vi "PR4000 cfg data.vi"(8 "error in (no error)":errorcluster, 10 "Channel parsed command info":T1, 11 "MKS4000b in":refnum<class "MKS4000b.lvclass">) -> (0 "error out":errorcluster, 2 "new commands":string, 3 "MKS4000b out":refnum<class "MKS4000b.lvclass">)   [LabVIEW 2013, in "MKS4000b.lvclass"]
uses:
  MKS4000b.lvclass
  Shared/Device Driver/channel parsed cmd cluster.ctl
  MKS4000b.lvclass/MKS4000b.ctl
  shared/CompressAndUpdate(Poly)/CompressAndUpdate(Numeric).vi
  shared/CompressAndUpdate(Poly)/CompressAndUpdate(Enum).vi
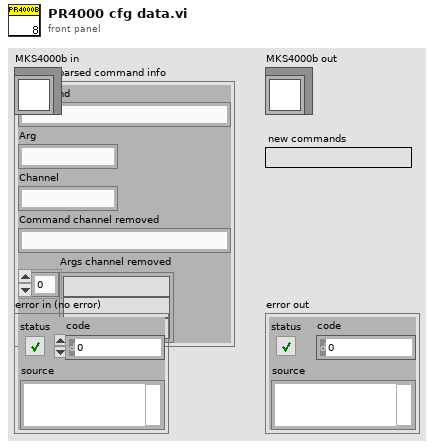
[diagram p1: front panel]
types:
  T1 = typedef "channel parsed cmd cluster.ctl" = cluster{"Command":string, "Arg":string, "Channel":string, "Command channel removed":string, "Args channel removed":string[]}
  T2 = typedef "channel_mode_typdef.ctl" = enum16{"Pressure", "Flow"}
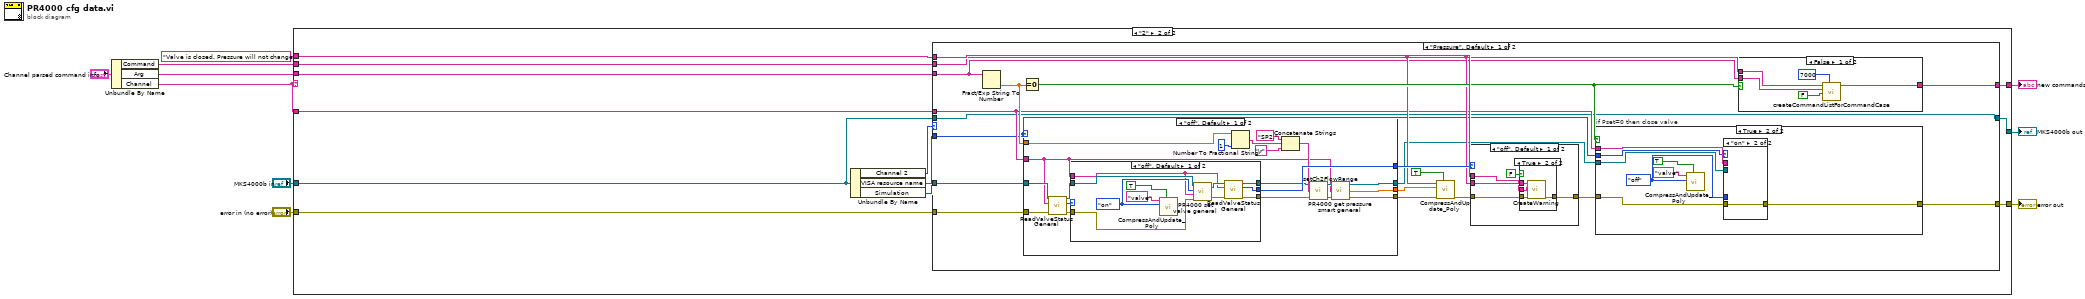
[diagram p0: block diagram]
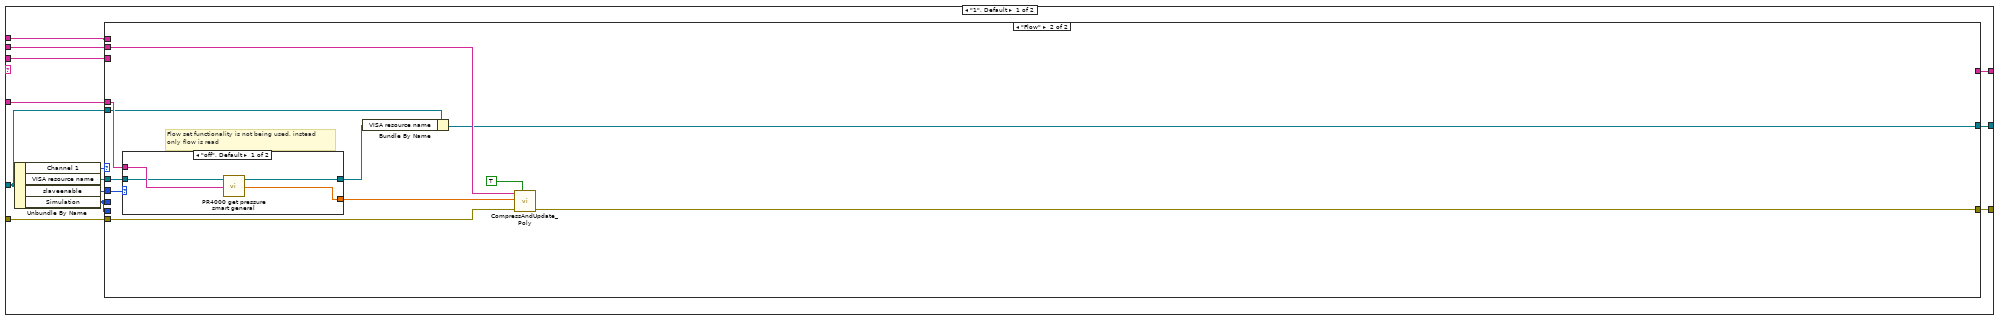
[diagram p2: hidden frame]
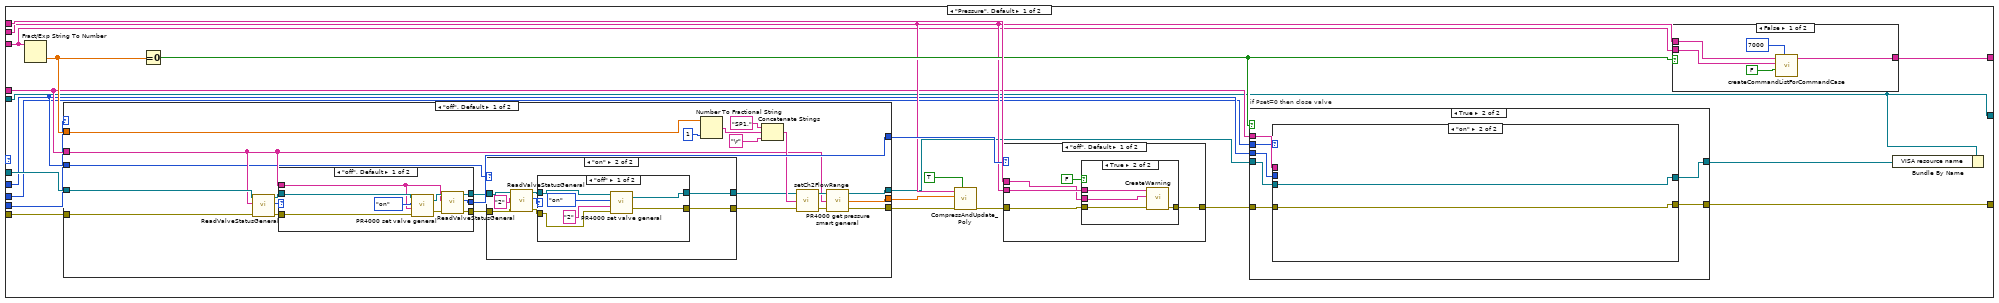
[diagram p3: hidden frame]
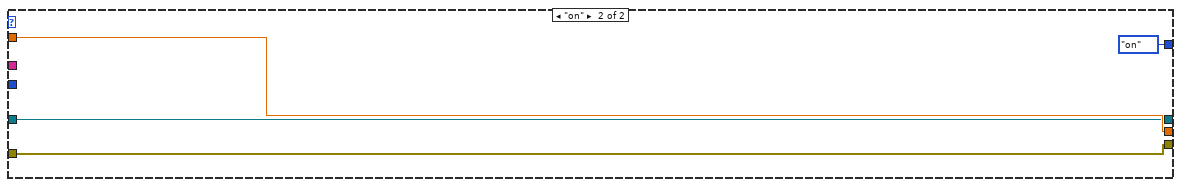
[diagram p7: hidden frame]
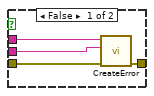
[diagram p9: hidden frame]
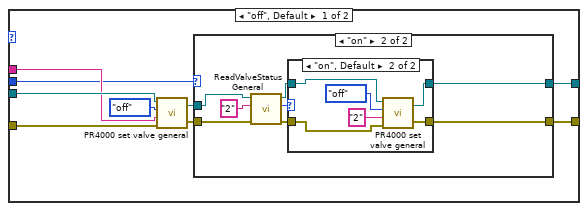
[diagram p12: hidden frame]
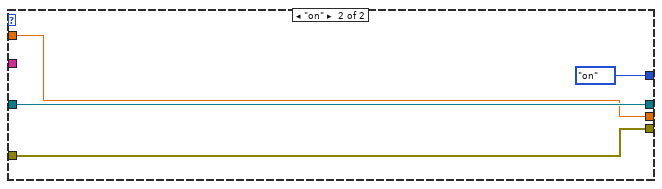
[diagram p17: hidden frame]
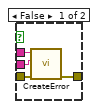
[diagram p19: hidden frame]
diagram:
  n1 = Unbundle By Name("Channel parsed command info") -> ("Command"=w9:string, "Arg"=w8:string, "Channel"=w7:string)
  n2 = case shown="\"2\"" w7 {
    tunnel: [w23 w187] -> w1
    tunnel: [w22 w186] -> w2
    tunnel: "Valve is closed. Pressure will not change!" ("error message (\"\")") -> [w21 w185]
    tunnel: "error in (no error)" -> [w20 w184]
    tunnel: [w19 w183] -> w4
    tunnel: "MKS4000b in" -> [w17 w181]
    tunnel: w9 -> [w18 w182]
    tunnel: w7 -> [w15 w179]
    tunnel: w8 -> [w13 w177]
    frame "1", Default {
      n3 = Unbundle By Name(w17) -> ("Channel 1"=w16:T2, "VISA resource name"=w14:refnum<visa-resource-name>, "slaveenable"=w12:enum16{"off", "on"}, "Simulation"=w11:enum16{"off", "on"})
      n4 = case shown="\"Flow\"" w16 {
        tunnel: [w27 w164] -> w23
        tunnel: [w45 _] -> w22
        tunnel: w21 -> [w43 _]
        tunnel: w20 -> [w35 w167]
        tunnel: [w39 w168] -> w19
        tunnel: w18 -> [w37 w169]
        tunnel: w17 -> [w27 w163]
        tunnel: w15 -> [w29 w166]
        tunnel: w14 -> [w36 w165]
        tunnel: w13 -> [w30 _]
        tunnel: w12 -> [w28 w160]
        tunnel: w11 -> [w25 _]
        tunnel: w11 -> [w24 _]
        frame "Pressure", Default {
          n5 = Fract/Exp String To Number(string=w30) -> (number=w34:dbl)  [unwired: 3 in, 1 out]
          n6 = case shown="\"off\", Default" w25 {
            tunnel: [w68 enum16{"off", "on"}."on" ("Settings.Save")] -> w41
            tunnel: w36 -> [w67 w101]
            tunnel: w35 -> [w66 w100]
            tunnel: w34 -> [w58 w102]
            tunnel: [w54 w100] -> w33
            tunnel: [w53 w102] -> w32
            tunnel: [w52 w101] -> w31
            tunnel: w29 -> [w51 _]
            tunnel: w28 -> [w46 _]
            frame "off", Default {
              n7 = call "ReadValveStatusGeneral.vi"("error in (no error)"=w66, "channel no in"=w51, "Comport PR4000"=w67) -> ("error out"=w65:errorcluster, "Settings.Save"=w64:enum16{"off", "on"}, "VISA resource name out"=w63:refnum<visa-resource-name>)  [unwired: 6 in]
              n8 = case shown="\"off\", Default" w64 {
                selector: w64 -> [_ w97]
                tunnel: [w87 w96] -> w50
                tunnel: w65 -> [w95 w98]
                tunnel: [w92 w98] -> w49
                tunnel: [w88 w97] -> w68
                tunnel: w63 -> [w93 w96]
                tunnel: w51 -> [w89 _]
                frame "off", Default {
                  n9 = call "PR4000 set valve general.vi"("error"=w95, "channel no in"=w89, "Settings.Valve"=enum16{"off", "on"}."on" ("Settings.Save"), "Comport PR4000"=w93) -> ("error out"=w91:errorcluster, "Comport PR4000 out"=w90:refnum<visa-resource-name>)
                  n10 = call "ReadValveStatusGeneral.vi"("error in (no error)"=w91, "channel no in"=w89, "Comport PR4000"=w90) -> ("error out"=w92:errorcluster, "Settings.Save"=w88:enum16{"off", "on"}, "VISA resource name out"=w87:refnum<visa-resource-name>)  [unwired: 6 in]
                }
                frame "on" {
                }
              }
              n11 = case shown="\"on\"" w46 {
                tunnel: w50 -> [w70 w78]
                tunnel: w49 -> [w69 w76]
                tunnel: [w70 w72] -> w48
                tunnel: [w69 w71] -> w47
                frame "off", Default {
                }
                frame "on" {
                  n12 = call "ReadValveStatusGeneral.vi"("error in (no error)"=w76, "channel no in"="2", "Comport PR4000"=w78) -> ("error out"=w73:errorcluster, "Settings.Save"=w75:enum16{"off", "on"}, "VISA resource name out"=w74:refnum<visa-resource-name>)  [unwired: 6 in]
                  n13 = case shown="\"off\"" w75 {
                    tunnel: w74 -> [w84 w86]
                    tunnel: [w83 w86] -> w72
                    tunnel: w73 -> [w82 w85]
                    tunnel: [w81 w85] -> w71
                    frame "off" {
                      n14 = call "PR4000 set valve general.vi"("error"=w82, "channel no in"="2", "Settings.Valve"=enum16{"off", "on"}."on", "Comport PR4000"=w84) -> ("error out"=w81:errorcluster, "Comport PR4000 out"=w83:refnum<visa-resource-name>)
                    }
                    frame "on", Default {
                    }
                  }
                }
              }
              n15 = Number To Fractional String(number=w58, precision (6)=i16 1) -> (F-format string=w60:string)  [unwired: 2 out]
              n16 = Concatenate Strings("SP1," ("string"), w60, "\r" ("string")) -> (w57:string)
              n17 = call "setCh2FlowRange.vi"("error"=w47, "command in"=w57, "Comport PR4000"=w48) -> ("error out"=w55:errorcluster, "VISA resource name out"=w56:refnum<visa-resource-name>)  [unwired: 1 out]
              n18 = call "PR4000 get pressure smart general.vi"("error in"=w55, "Channel in"=w51, "Comport PR4000"=w56) -> ("error out"=w54:errorcluster, "Actual"=w53:dbl, "VISA Refnum out"=w52:refnum<visa-resource-name>)
            }
            frame "on" {
            }
          }
          n19 = Equal To 0?(x=w34) -> (x = 0?=w38:bool)
          n20 = call-poly "CompressAndUpdate_Poly.vi"("force CVT update (false)"=TRUE ("force CVT update"), "error in"=w33, "Numeric"=w32, "command or variable name"=w37) -> ("error out"=w42:errorcluster)  [unwired: 7 in]
          n21 = case shown="\"off\", Default" w41 {
            tunnel: w42 -> [w112 w121]
            tunnel: [w111 w121] -> w40
            tunnel: w37 -> [w110 _]
            tunnel: w43 -> [w109 _]
            frame "off", Default {
              n22 = case shown="True" FALSE {
                tunnel: w112 -> [w114 w120]
                tunnel: [w113 w119] -> w111
                tunnel: w110 -> [w116 w118]
                tunnel: w109 -> [w115 w117]
                frame False {
                  n23 = call "CreateError.vi"("user error in"=w114, "error message (\"\")"=w115, "command"=w116) -> ("user error  out"=w113:errorcluster)  [unwired: 8 in]
                }
                frame True {
                  n24 = call "CreateWarning.vi"("user error in"=w120, "error message (\"\")"=w117, "command"=w118) -> ("user error  out"=w119:errorcluster)  [unwired: 8 in]
                }
              }
            }
            frame "on" {
            }
          }
          n25 = case "if Pset=0 then close valve" shown="True" w38 {
            tunnel: w40 -> [w123 w130]
            tunnel: [w123 w125] -> w39
            tunnel: w31 -> [w122 w129]
            tunnel: w29 -> [_ w128]
            tunnel: w28 -> [_ w127]
            tunnel: [w122 w126] -> w26
            tunnel: w24 -> [_ w124]
            frame False {
            }
            frame True {
              n26 = case shown="\"on\"" w124 {
                tunnel: w130 -> [w139 w158]
                tunnel: w129 -> [w138 w159]
                tunnel: w128 -> [w137 _]
                tunnel: w127 -> [w136 _]
                tunnel: [w132 w159] -> w126
                tunnel: [w131 w158] -> w125
                frame "off", Default {
                  n27 = call "PR4000 set valve general.vi"("error"=w139, "channel no in"=w137, "Settings.Valve"=enum16{"off", "on"}."off" ("Settings.Save"), "Comport PR4000"=w138) -> ("error out"=w135:errorcluster, "Comport PR4000 out"=w133:refnum<visa-resource-name>)
                  n28 = case shown="\"on\"" w136 {
                    tunnel: w135 -> [w141 w148]
                    tunnel: [w140 w144] -> w132
                    tunnel: [w141 w143] -> w131
                    tunnel: w133 -> [w140 w142]
                    frame "off", Default {
                    }
                    frame "on" {
                      n29 = call "ReadValveStatusGeneral.vi"("error in (no error)"=w148, "channel no in"="2", "Comport PR4000"=w142) -> ("error out"=w145:errorcluster, "Settings.Save"=w147:enum16{"off", "on"}, "VISA resource name out"=w146:refnum<visa-resource-name>)  [unwired: 6 in]
                      n30 = case shown="\"on\", Default" w147 {
                        tunnel: w146 -> [w151 w157]
                        tunnel: [w151 w156] -> w144
                        tunnel: w145 -> [w150 w155]
                        tunnel: [w150 w154] -> w143
                        frame "off" {
                        }
                        frame "on", Default {
                          n31 = call "PR4000 set valve general.vi"("error"=w155, "channel no in"="2", "Settings.Valve"=enum16{"off", "on"}."off", "Comport PR4000"=w157) -> ("error out"=w154:errorcluster, "Comport PR4000 out"=w156:refnum<visa-resource-name>)
                        }
                      }
                    }
                  }
                }
                frame "on" {
                }
              }
            }
          }
          n32 = case shown="False" w38 {
            tunnel: w30 -> [w107 _]
            tunnel: [w105 _] -> w45
            tunnel: w37 -> [w104 _]
            frame False {
              n33 = call "createCommandListForCommandCase.vi"("timeout (optional)"=7000, "immediate Check (only once)"=FALSE, "setvalue"=w107, "command"=w104) -> ("new commands"=w105:string)  [unwired: 7 in]
            }
            frame True {
            }
          }
          n34 = Bundle By Name(cluster=w27, "VISA resource name"=w26) -> ()  [unwired: 1 out]
        }
        frame "Flow" {
          # "Flow set functionality is not being used, instead\nonly flow is read"
          n35 = case shown="\"off\", Default" w160 {
            tunnel: w166 -> [w174 _]
            tunnel: w165 -> [w173 w175]
            tunnel: [w172 _] -> w162
            tunnel: [w171 w175] -> w161
            frame "off", Default {
              n36 = call "PR4000 get pressure smart general.vi"("Channel in"=w174, "Comport PR4000"=w173) -> ("Actual"=w172:dbl, "VISA Refnum out"=w171:refnum<visa-resource-name>)  [unwired: 1 in, 1 out]
            }
            frame "on" {
            }
          }
          n37 = Bundle By Name(cluster=w163, "VISA resource name"=w161) -> (w164:refnum<class "MKS4000b.lvclass">)
          n38 = call-poly "CompressAndUpdate_Poly.vi"("force CVT update (false)"=TRUE ("force CVT update"), "error in"=w167, "Numeric"=w162, "command or variable name"=w169) -> ("error out"=w168:errorcluster)  [unwired: 7 in]
        }
      }
    }
    frame "2" {
      n39 = Unbundle By Name(w181) -> ("Channel 2"=w180:T2, "VISA resource name"=w178:refnum<visa-resource-name>, "Simulation"=w176:enum16{"off", "on"})
      n40 = case shown="\"Pressure\", Default" w180 {
        tunnel: [w189 w285] -> w187
        tunnel: [w206 _] -> w186
        tunnel: w185 -> [w204 _]
        tunnel: w184 -> [w196 w281]
        tunnel: [w200 w288] -> w183
        tunnel: w182 -> [w198 w289]
        tunnel: w181 -> [w189 w284]
        tunnel: w179 -> [w190 w287]
        tunnel: w178 -> [w197 w286]
        tunnel: w177 -> [w191 _]
        tunnel: w176 -> [w188 w279]
        frame "Pressure", Default {
          n41 = Fract/Exp String To Number(string=w191) -> (number=w195:dbl)  [unwired: 3 in, 1 out]
          n42 = Equal To 0?(x=w195) -> (x = 0?=w199:bool)
          n43 = case shown="\"off\", Default" w188 {
            tunnel: [w226 enum16{"off", "on"}."on" ("Settings.Save")] -> w202
            tunnel: w197 -> [w225 w244]
            tunnel: w196 -> [w224 w243]
            tunnel: w195 -> [w216 w241]
            tunnel: [w210 w243] -> w194
            tunnel: [w209 w241] -> w193
            tunnel: [w208 w244] -> w192
            tunnel: w190 -> [w207 _]
            frame "off", Default {
              n44 = call "ReadValveStatusGeneral.vi"("error in (no error)"=w224, "channel no in"=w207, "Comport PR4000"=w225) -> ("error out"=w223:errorcluster, "Settings.Save"=w222:enum16{"off", "on"}, "VISA resource name out"=w221:refnum<visa-resource-name>)  [unwired: 6 in]
              n45 = case shown="\"off\", Default" w222 {
                selector: w222 -> [_ w239]
                tunnel: [w227 w238] -> w213
                tunnel: w223 -> [w237 w240]
                tunnel: [w232 w240] -> w214
                tunnel: [w228 w239] -> w226
                tunnel: w221 -> [w233 w238]
                tunnel: w207 -> [w229 _]
                frame "off", Default {
                  w235 = enum16{"off", "on"}."on" ("Settings.Save")
                  n46 = call-poly "CompressAndUpdate_Poly.vi"("force CVT update (false)"=TRUE, "enum variant"=w235, "command or variable name"="valve") -> ()  [unwired: 8 in, 1 out]
                  n47 = call "PR4000 set valve general.vi"("error"=w237, "channel no in"=w229, "Settings.Valve"=w235, "Comport PR4000"=w233) -> ("error out"=w231:errorcluster, "Comport PR4000 out"=w230:refnum<visa-resource-name>)
                  n48 = call "ReadValveStatusGeneral.vi"("error in (no error)"=w231, "channel no in"=w229, "Comport PR4000"=w230) -> ("error out"=w232:errorcluster, "Settings.Save"=w228:enum16{"off", "on"}, "VISA resource name out"=w227:refnum<visa-resource-name>)  [unwired: 6 in]
                }
                frame "on" {
                }
              }
              n49 = Number To Fractional String(number=w216, precision (6)=i16 1) -> (F-format string=w218:string)  [unwired: 2 out]
              n50 = Concatenate Strings("SP2," ("string"), w218, "\r" ("string")) -> (w215:string)
              n51 = call "setCh2FlowRange.vi"("error"=w214, "command in"=w215, "Comport PR4000"=w213) -> ("error out"=w211:errorcluster, "VISA resource name out"=w212:refnum<visa-resource-name>)  [unwired: 1 out]
              n52 = call "PR4000 get pressure smart general.vi"("error in"=w211, "Channel in"=w207, "Comport PR4000"=w212) -> ("error out"=w210:errorcluster, "Actual"=w209:dbl, "VISA Refnum out"=w208:refnum<visa-resource-name>)
            }
            frame "on" {
            }
          }
          n53 = call-poly "CompressAndUpdate_Poly.vi"("force CVT update (false)"=TRUE ("force CVT update"), "error in"=w194, "Numeric"=w193, "command or variable name"=w198) -> ("error out"=w203:errorcluster)  [unwired: 7 in]
          n54 = case shown="\"off\", Default" w202 {
            tunnel: w203 -> [w254 w263]
            tunnel: [w253 w263] -> w201
            tunnel: w198 -> [w252 _]
            tunnel: w204 -> [w251 _]
            frame "off", Default {
              n55 = case shown="True" FALSE {
                tunnel: w254 -> [w256 w262]
                tunnel: [w255 w261] -> w253
                tunnel: w252 -> [w258 w260]
                tunnel: w251 -> [w257 w259]
                frame False {
                  n56 = call "CreateError.vi"("user error in"=w256, "error message (\"\")"=w257, "command"=w258) -> ("user error  out"=w255:errorcluster)  [unwired: 8 in]
                }
                frame True {
                  n57 = call "CreateWarning.vi"("user error in"=w262, "error message (\"\")"=w259, "command"=w260) -> ("user error  out"=w261:errorcluster)  [unwired: 8 in]
                }
              }
            }
            frame "on" {
            }
          }
          n58 = case "if Pset=0 then close valve" shown="True" w199 {
            tunnel: w201 -> [w264 w269]
            tunnel: [w264 w268] -> w200
            tunnel: w192 -> [_ w267]
            tunnel: w190 -> [_ w266]
            tunnel: w188 -> [_ w265]
            frame False {
            }
            frame True {
              w271 = enum16{"off", "on"}."off" ("Settings.Save")
              n59 = call-poly "CompressAndUpdate_Poly.vi"("force CVT update (false)"=TRUE, "enum variant"=w271, "command or variable name"="valve") -> ()  [unwired: 8 in, 1 out]
              n60 = case shown="\"on\"" w265 {
                tunnel: w271 -> [w277 _]
                tunnel: w269 -> [w276 w278]
                tunnel: [w275 w278] -> w268
                tunnel: w267 -> [w274 _]
                tunnel: w266 -> [w273 _]
                frame "off", Default {
                  n61 = call "PR4000 set valve general.vi"("error"=w276, "channel no in"=w273, "Settings.Valve"=w277, "Comport PR4000"=w274) -> ("error out"=w275:errorcluster)  [unwired: 1 out]
                }
                frame "on" {
                }
              }
            }
          }
          n62 = case shown="False" w199 {
            tunnel: w191 -> [w249 _]
            tunnel: [w247 _] -> w206
            tunnel: w198 -> [w246 _]
            frame False {
              n63 = call "createCommandListForCommandCase.vi"("timeout (optional)"=7000, "immediate Check (only once)"=FALSE, "setvalue"=w249, "command"=w246) -> ("new commands"=w247:string)  [unwired: 7 in]
            }
            frame True {
            }
          }
        }
        frame "Flow" {
          # "Flow set functionality is not being used, instead\nonly flow is read"
          n64 = case shown="\"on\"" w279 {
            tunnel: w287 -> [w296 _]
            tunnel: w286 -> [w295 w297]
            tunnel: [w294 0.0 ("Actual")] -> w283
            tunnel: [w293 w297] -> w282
            tunnel: w281 -> [w292 w298]
            tunnel: [w291 w298] -> w280
            frame "off", Default {
              n65 = call "PR4000 get pressure smart general.vi"("error in"=w292, "Channel in"=w296, "Comport PR4000"=w295) -> ("error out"=w291:errorcluster, "Actual"=w294:dbl, "VISA Refnum out"=w293:refnum<visa-resource-name>)
            }
            frame "on" {
            }
          }
          n66 = Bundle By Name(cluster=w284, "VISA resource name"=w282) -> (w285:refnum<class "MKS4000b.lvclass">)
          n67 = call-poly "CompressAndUpdate_Poly.vi"("force CVT update (false)"=TRUE ("force CVT update"), "error in"=w280, "Numeric"=w283, "command or variable name"=w289) -> ("error out"=w288:errorcluster)  [unwired: 7 in]
        }
      }
    }
  }
  "error out" <- w4
  "new commands" <- w2
  "MKS4000b out" <- w1
